vi "Group Channels By VS and MB Type.vi"(7 "Channel Type":T1, 8 "error in (no error)":errorcluster, 11 "Item Ref in":T2 format="%.0x") -> (0 "error out":errorcluster, 2 "Channels":T3 {"Holding Registers"."Mapping"."VS Reference" format="%.0x"; "Input Registers"."Mapping"."VS Reference" format="%.0x"; "Discrete Inputs"."Mapping"."VS Reference" format="%.0x"; "Coils"."Mapping"."VS Reference" format="%.0x"}, 3 "Device Ref out":T2 format="%.0x")   [LabVIEW 2021, in "Modbus Master System Explorer.lvlib"]
uses:
  Modbus Master System Explorer.lvlib
  Shared/Controls/Data Model/Channel Data.ctl
  Shared/Controls/Data Model/Channel.ctl
  SubVIs/Modbus Type.ctl
  <vilib>/NI VeriStand/Custom Device API/Custom Device Channel Type.ctl
  Shared/Controls/Data Model/Mapping.ctl
  Shared/Controls/Data Model/DataType.ctl
  <vilib>/NI VeriStand/Custom Device API/Custom Device Item Ref.ctl
  <vilib>/NI VeriStand/Custom Device API/Custom Device API.lvlib
  Shared/Modbus Master Shared.lvlib
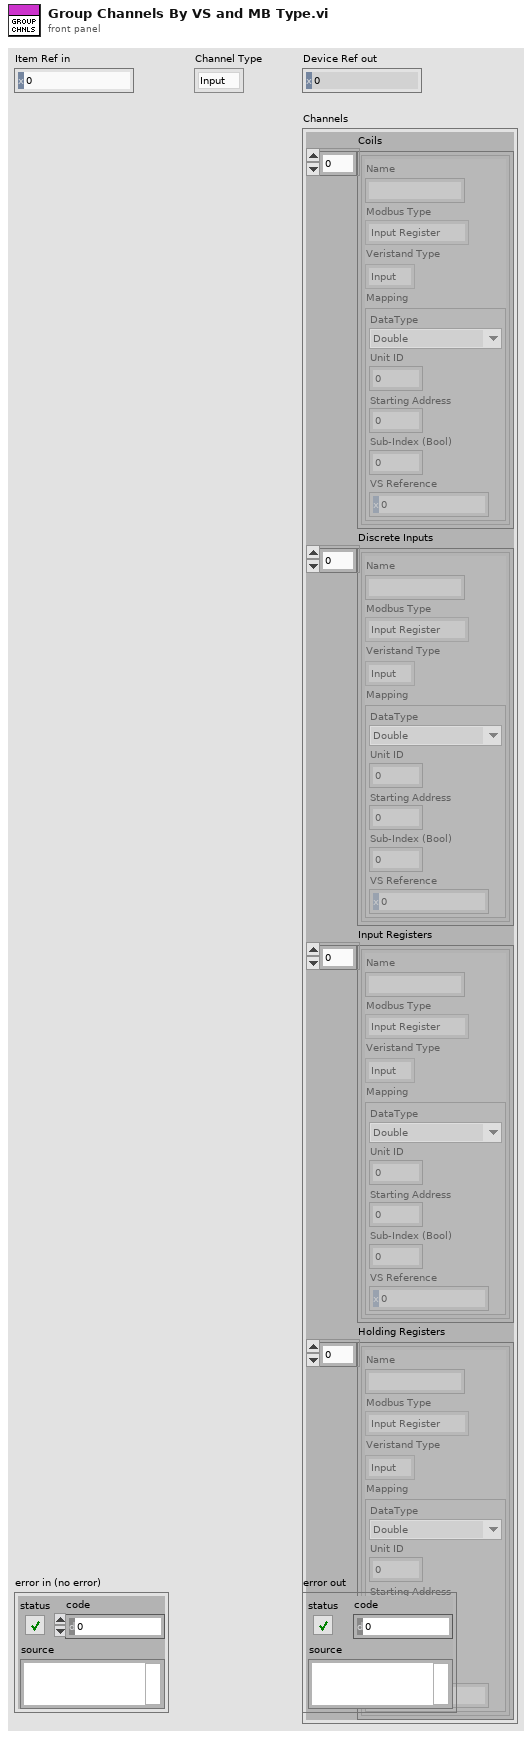
[diagram p1: front panel]
types:
  T1 = typedef "Custom Device API.lvlib/Custom Device Channel Type.ctl" = enum16{"Input", "Output"}
  T2 = typedef "Custom Device API.lvlib/Custom Device Item Ref.ctl" = u64
  T3 = typedef "Modbus Master Shared.lvlib/Channel Data.ctl" = cluster{"Coils":T4[], "Discrete Inputs":T4[], "Input Registers":T4[], "Holding Registers":T4[]}
  T4 = typedef "Modbus Master Shared.lvlib/Channel.ctl" = cluster{"Name":string, "Modbus Type":T5, "Veristand Type":T1, "Mapping":T6}
  T5 = typedef "Modbus Master Shared.lvlib/Modbus Type.ctl" = enum16{"Coil", "Discrete Input", "Holding Register", "Input Register"}
  T6 = typedef "Modbus Master Shared.lvlib/Mapping.ctl" = cluster{"DataType":T7, "Unit ID":u8, "Starting Address":u16, "Sub-Index (Bool)":u16, "VS Reference":T2}
  T7 = typedef "Modbus Master Shared.lvlib/DataType.ctl" = enum16{"Double", "Single", "I64", "I32", "I16", "I8", "U64", "U32", "U16", "U8", "Boolean"}
  T8 = typedef "Custom Device API.lvlib/Custom Device Item Info.ctl" = cluster{"Name":string, "Is Channel":bool, "GUID":string, "Is Waveform":bool}
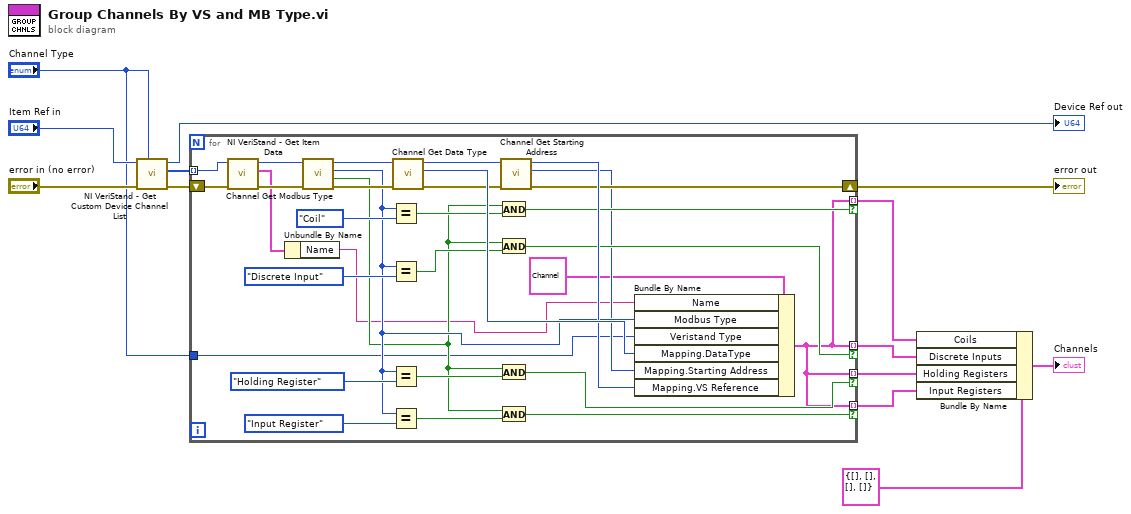
[diagram p0: block diagram]
diagram:
  n1 = call <vilib>:"NI VeriStand - Get Custom Device Channel List.vi"("Channel Type"="Channel Type", "error in (no error)"="error in (no error)", "Device Ref in"="Item Ref in") -> ("error out"=w3:errorcluster, "Specified Channel Ref List"=w1:T2[], "Device Ref out"=→"Device Ref out":T2)  [unwired: 6 in]
  n2 = for {
    tunnel: w1 -> [w16] mode=indexing
    tunnel: "Channel Type" -> [w17]
    tunnel: [w24] -> w10 mode=indexing if=w30
    tunnel: [w24] -> w11 mode=indexing if=w29
    tunnel: [w24] -> w12 mode=indexing if=w28
    tunnel: [w24] -> w13 mode=indexing if=w27
    shift-right: [w33] -> w8
    shift-left: w3 -> [w21]
    n3 = call <vilib>:"NI VeriStand - Get Item Data.vi"("error in (no error)"=w21, "Item Ref in"=w16) -> ("error out"=w20:errorcluster, "Item Info"=w19:T8, "Item Ref out"=w15:T2)  [unwired: 6 in, 1 out]
    n4 = Unbundle By Name(w19) -> ("Name"=w18:string)
    n5 = call "Channel Get Modbus Type.vi"("error in (no error)"=w20, "Channel Ref"=w15) -> ("error out"=w41:errorcluster, "Is MB Type?"=w26:bool, "Type"=w32:T5, "Item Ref out"=w44:T2)  [unwired: 6 in]
    n6 = Equal?(x=w32, y=Modbus_Type."Coil") -> (x = y?=w31:bool)
    n7 = Equal?(x=w32, y=Modbus_Type."Discrete Input") -> (x = y?=w36:bool)
    n8 = Equal?(x=w32, y=Modbus_Type."Holding Register") -> (x = y?=w35:bool)
    n9 = Equal?(x=w32, y=Modbus_Type."Input Register") -> (x = y?=w34:bool)
    n10 = call "Channel Get Data Type.vi"("error in (no error)"=w41, "Item Ref in"=w44) -> ("error out"=w23:errorcluster, "Data Type"=w43:T7, "Item Ref out"=w22:T2)  [unwired: 7 in]
    n11 = And(x=w26, y=w31) -> (x .and. y?=w30:bool)
    n12 = And(x=w26, y=w36) -> (x .and. y?=w29:bool)
    n13 = And(x=w26, y=w35) -> (x .and. y?=w28:bool)
    n14 = And(x=w26, y=w34) -> (x .and. y?=w27:bool)
    n15 = call "Channel Get Starting Address.vi"("error in (no error)"=w23, "Item Ref in"=w22) -> ("error out"=w33:errorcluster, "Value"=w25:u16, "Item Ref out"=w42:T2)  [unwired: 7 in]
    n16 = Bundle By Name(cluster=T4 {"Name"="", "Modbus Type"=enum."Input Register", "Veristand Type"=enum."Output", "Mapping"={"DataType"=enum."Double", "Unit ID"=0, "Starting Address"=0, "Sub-Index (Bool)"=0, "VS Reference"=0}} ("Channel"), "Name"=w18, "Modbus Type"=w32, "Veristand Type"=w17, "Mapping.DataType"=w43, "Mapping.Starting Address"=w25, "Mapping.VS Reference"=w42) -> (w24:T4)
  }
  "error out" <- w8
  n17 = Bundle By Name(cluster=T3 {"Coils"=[], "Discrete Inputs"=[], "Input Registers"=[], "Holding Registers"=[]} ("Outputs"), "Coils"=w10, "Discrete Inputs"=w11, "Holding Registers"=w12, "Input Registers"=w13) -> (→"Channels":T3)
